vi "Keithley DMM6500 DAQ6500 Series General Scanning.vi"() -> ()   [LabVIEW 2020]
doc: "This example shows how to configure a measurement and take multiple readings."
uses:
  <instrlib>/Keithley DMM6500 DAQ6500 Series/Public/Data/Read (Multiple Points).vi
  <instrlib>/Keithley DMM6500 DAQ6500 Series/Keithley DMM6500 DAQ6500 Series.lvlib
panel:
  in  "Buffer Element1 ()":i32(ring) items=["", "Date", "Extra", "Formatted", "Fractional", "Reading", "Relative", "Seconds", "Status", "Time", "Tstamp", "Unit", "CHAN", "Extra Format", "Extra Unit"]
  in  "Buffer Element2 ()":i32(ring) items=["", "Date", "Extra", "Formatted", "Fractional", "Reading", "Relative", "Seconds", "Status", "Time", "Tstamp", "Unit", "CHAN", "Extra Form", "Extra Unit"]
  out "Measurements":dbl[](array[numeric])
  in  "Auto Zero (0: Enable)":u32(ring) items=["Enable", "Disable", "Once"]
  in  "Buffer Size (10)":u32=10
  in  "Enable Limit (F: Disable)":bool
  in  "Upper Limit (0)":dbl
  in  "Limit Number (1: Limit 1)":i32(ring)=1 items=["Limit 1"=1, "Limit 2"=2]
  in  "Lower Limit (0)":dbl
  in  "Scan Interval (60 s)":dbl=60.0
  in  "Scan Count (1)":u32=1
  in  "Reading Buffer (\"defbuffer1\")":string="defbuffer1"
  in  "Auto Range (T: Enable)":bool=TRUE
  in  "Function (0: Voltage DC)":i32(ring) items=[" Voltage DC", "Voltage AC", "Current DC", "Current AC", "Resistance", "4-wire Resistance", "Diode", "Capacitance", "Temperature", "Continuity", "Frequency", "Period", "Voltage Ratio", "Digitize Voltage", "Digitize Current"]
  in  "Manual Range (0)":dbl
  in  "Channel List (\"2:10\")":string="2:10"
  in  "VISA resource name":refnum<visa-resource-name>
  # "(c) 2018-2022 National Instruments.  ALL RIGHTS RESERVED."
  # "This example VI demonstrates setting up basic scans on either the DAQ6500 or DMM6500 Series."
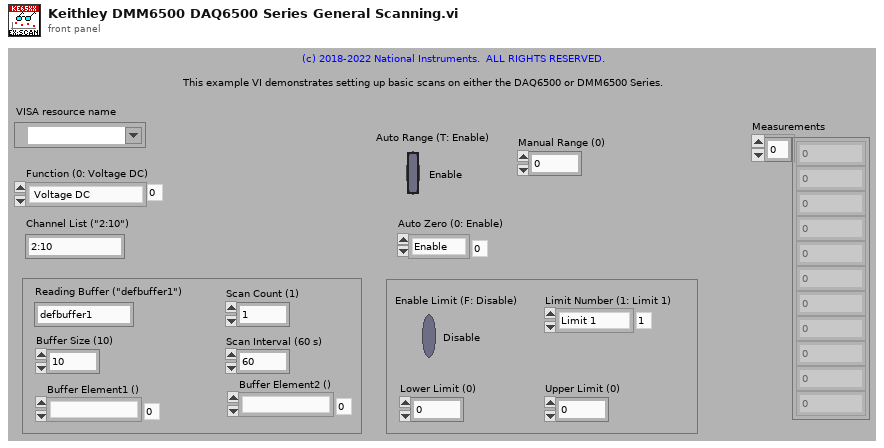
[diagram p1: front panel]
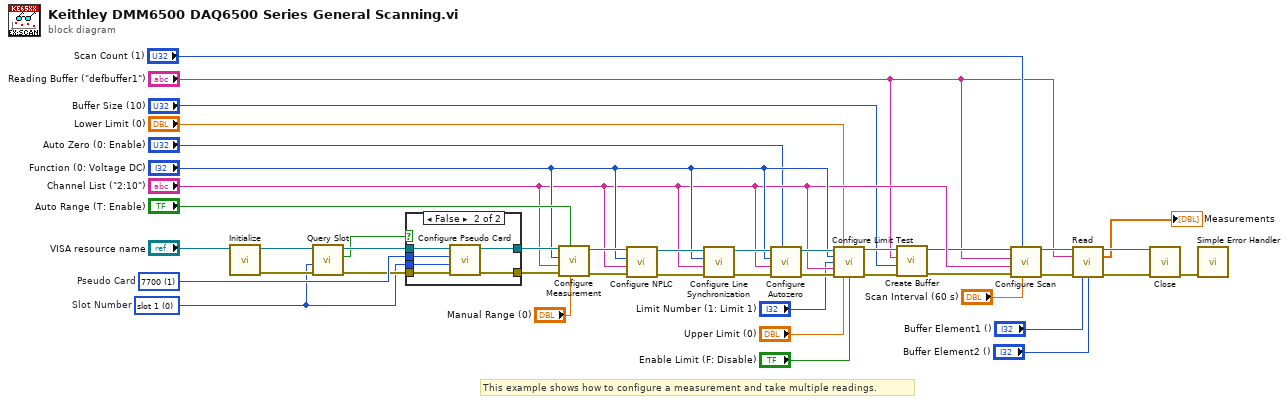
[diagram p0: block diagram]
diagram:
  w4 = 0 items=["slot 1", "slot 2"]  # Slot Number
  w8 = 1 items=["0", "7700", "7701", "7702", "7703", "7705", "7706", "7707", "7708", "7709", "7710", "7711", "7712"]  # Pseudo Card
  # "This example shows how to configure a measurement and take multiple readings."
  n1 = call <instrlib>:"Initialize.vi"("VISA resource name"="VISA resource name") -> ("error out"=w6:errorcluster, "VISA resource name out"=w41:refnum<visa-resource-name>)  [unwired: 9 in]
  n2 = call <instrlib>:"Query Slot.vi"("error in (no error)"=w6, "Slot Number(0: slot 1)"=w4, "VISA resource name"=w41) -> ("error out"=w5:errorcluster, "Real Card In Slot"=w3:bool, "VISA resource name out"=w7:refnum<visa-resource-name>)  [unwired: 6 in]
  n3 = case shown="False" w3 {
    tunnel: [w45 w51] -> w40
    tunnel: [w44 w50] -> w39
    tunnel: w8 -> [_ w49]
    tunnel: w7 -> [w45 w48]
    tunnel: w5 -> [w44 w47]
    tunnel: w4 -> [_ w46]
    frame True {
    }
    frame False {
      n4 = call <instrlib>:"Configure Pseudo Card.vi"("error in (no error)"=w47, "Slot Number (0: slot1)"=w46, "Pseudo Card (0:No pseudocard)"=w49, "VISA resource name"=w48) -> ("error out"=w50:errorcluster, "VISA resource name out"=w51:refnum<visa-resource-name>)  [unwired: 6 in]
    }
  }
  n5 = call <instrlib>:"Configure Measurement.vi"("Manual Range (1)"="Manual Range (0)", "Auto Range (T: Enable)"="Auto Range (T: Enable)", "error in (no error)"=w39, "Channel List(\"\")"="Channel List (\"2:10\")", "Function (0: Voltage DC)"="Function (0: Voltage DC)", "VISA resource name"=w40) -> ("error out"=w35:errorcluster, "VISA resource name out"=w36:refnum<visa-resource-name>)  [unwired: 4 in]
  n6 = call <instrlib>:"Configure NPLC.vi"("error in (no error)"=w35, "Channel List(\"\")"="Channel List (\"2:10\")", "Function (0: Voltage DC)"="Function (0: Voltage DC)", "VISA resource name"=w36) -> ("error out"=w33:errorcluster, "VISA resource name out"=w34:refnum<visa-resource-name>)  [unwired: 6 in]
  n7 = call <instrlib>:"Configure Line Synchronization.vi"("error in (no error)"=w33, "Channel List(\"\")"="Channel List (\"2:10\")", "Function (0: Voltage DC)"="Function (0: Voltage DC)", "VISA resource name"=w34) -> ("error out"=w31:errorcluster, "VISA resource name out"=w32:refnum<visa-resource-name>)  [unwired: 6 in]
  n8 = call <instrlib>:"Configure Autozero.vi"("Auto Zero (0: Enable)"="Auto Zero (0: Enable)", "error in (no error)"=w31, "Channel List(\"\")"="Channel List (\"2:10\")", "Function (0: Voltage DC)"="Function (0: Voltage DC)", "VISA resource name"=w32) -> ("error out"=w29:errorcluster, "VISA resource name out"=w30:refnum<visa-resource-name>)  [unwired: 5 in]
  n9 = call <instrlib>:"Configure Limit Test.vi"("VISA resource name"=w30, "Lower Limit (0)"="Lower Limit (0)", "Function (0: Voltage DC)"="Function (0: Voltage DC)", "Limit Number (1: Limit 1)"="Limit Number (1: Limit 1)", "Channel List(\"\")"="Channel List (\"2:10\")", "error in (no error)"=w29, "Upper Limit (0)"="Upper Limit (0)", "Enable Limit (F: Disable)"="Enable Limit (F: Disable)") -> ("VISA resource name out"=w15:refnum<visa-resource-name>, "error out"=w13:errorcluster)  [unwired: 6 in]
  n10 = call <instrlib>:"Create Buffer.vi"("error in (no error)"=w13, "Buffer Size (10)"="Buffer Size (10)", "Buffer Name (\"\")"="Reading Buffer (\"defbuffer1\")", "VISA resource name"=w15) -> ("error out"=w12:errorcluster, "VISA resource name out"=w14:refnum<visa-resource-name>)  [unwired: 6 in]
  n11 = call <instrlib>:"Configure Scan.vi"("Delay Seconds (0 s)"="Scan Interval (60 s)", "Scan Count (1)"="Scan Count (1)", "error in (no error)"=w12, "Channel List(\"\")"="Channel List (\"2:10\")", "Reading Buffer (\"\")"="Reading Buffer (\"defbuffer1\")", "VISA resource name"=w14) -> ("error out"=w17:errorcluster, "VISA resource name out"=w16:refnum<visa-resource-name>)  [unwired: 4 in]
  n12 = call-poly <instrlib>:"Read.vi"("VISA resource name"=w16, "Buffer Name (\"\")"="Reading Buffer (\"defbuffer1\")", "error in (no error)"=w17, "Buffer Element1 ()"="Buffer Element1 ()", "Buffer Element2 ()"="Buffer Element2 ()") -> ("VISA resource name out"=w20:refnum<visa-resource-name>, "Measurements"=→"Measurements":dbl[], "error out"=w19:errorcluster)  [unwired: 8 in]
  n13 = call <instrlib>:"Close.vi"("error in (no error)"=w19, "VISA resource name"=w20) -> ("error out"=w43:errorcluster)  [unwired: 9 in]
  n14 = call <vilib>:"Simple Error Handler.vi"("error in (no error)"=w43) -> ()  [unwired: 4 in, 5 out]
